vi "Disconnect.vi"(0 "object in":refnum<class "Laser_Ethernet.lvclass">, 5 "error in (no error)":errorcluster) -> (14 "object out":refnum<class "Laser_Ethernet.lvclass">, 19 "error out":errorcluster)   [LabVIEW 2023, in "Laser_Ethernet.lvclass"]
uses:
  Laser_Ethernet.lvclass
  Laser_Ethernet.lvclass/Laser_Ethernet.ctl
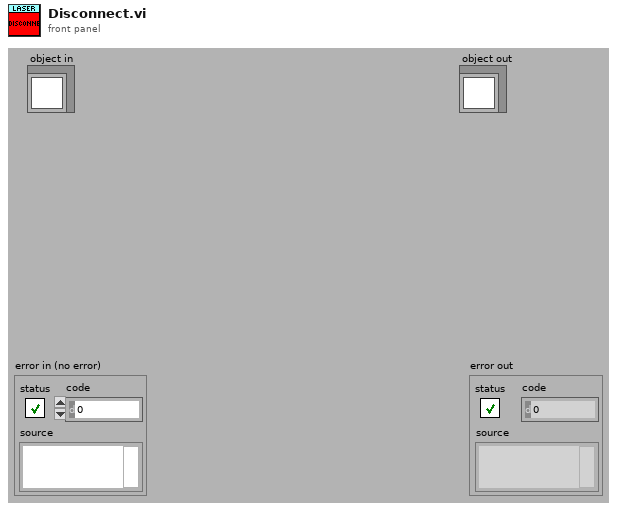
[diagram p1: front panel]
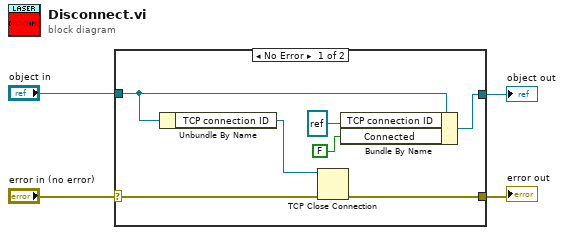
[diagram p0: block diagram]
diagram:
  n1 = case shown="No Error" "error in (no error)" {
    selector: "error in (no error)" -> [w6 w13]
    tunnel: [w5 w13] -> w3
    tunnel: [w10 w12] -> w1
    tunnel: "object in" -> [w11 w12]
    frame No Error {
      n2 = Unbundle By Name(w11) -> ("TCP connection ID"=w9:refnum<k5>)
      n3 = TCP Close Connection(connection ID=w9, error in (no error)=w6) -> (error out=w5:errorcluster)  [unwired: 1 in, 1 out]
      n4 = Bundle By Name(cluster=w11, "TCP connection ID"=refnum<k5> refnum, "Connected"=FALSE) -> (w10:refnum<class "Laser_Ethernet.lvclass">)
    }
    frame Error {
    }
  }
  "error out" <- w3
  "object out" <- w1
